vi "Test Save Animated GIF (Memory).vi"(8 "error in (no error)":errorcluster) -> (0 "error out":errorcluster, 3 "Pass?":bool)   [LabVIEW 2020]
uses:
  G-Image/Image IO/Controls/Dither Type.ctl
  G-Image/G-Image.lvlib
  0f1b1910-5d7c-4507-bdef-12e0c9c3451f.vi
  G-Image/Image IO/Polymorphic VIs/Save Animated GIF Image (Memory).vi
  G-Image/Image IO/Polymorphic VIs/Load Animated GIF Image (Memory).vi
panel:
  out "Waveform Chart":cluster{dbl, dbl}(graph)={-0.06975647374412564, 0.4806308479691592}
  out "Array":cluster{string, "new picture":picture}[](array[cluster])
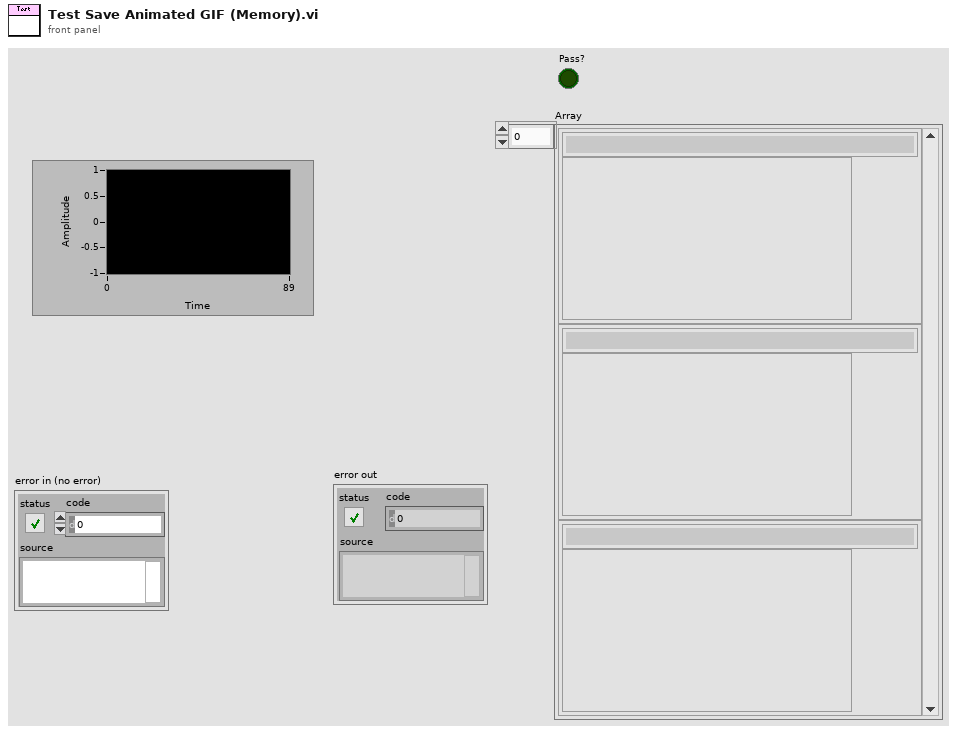
[diagram p1: front panel]
types:
  T1 = typedef "G-Image.lvlib/Dither Type.ctl" = enum32{"None", "Floyd-Steinberg"}
  T2 = typedef "imagedata.ctl" = cluster{"image type":i32, "image depth":i32, "image":u8[], "mask":u8[], "colors":u32[], "Rectangle":cluster{"left":i16, "top":i16, "right":i16, "bottom":i16}}
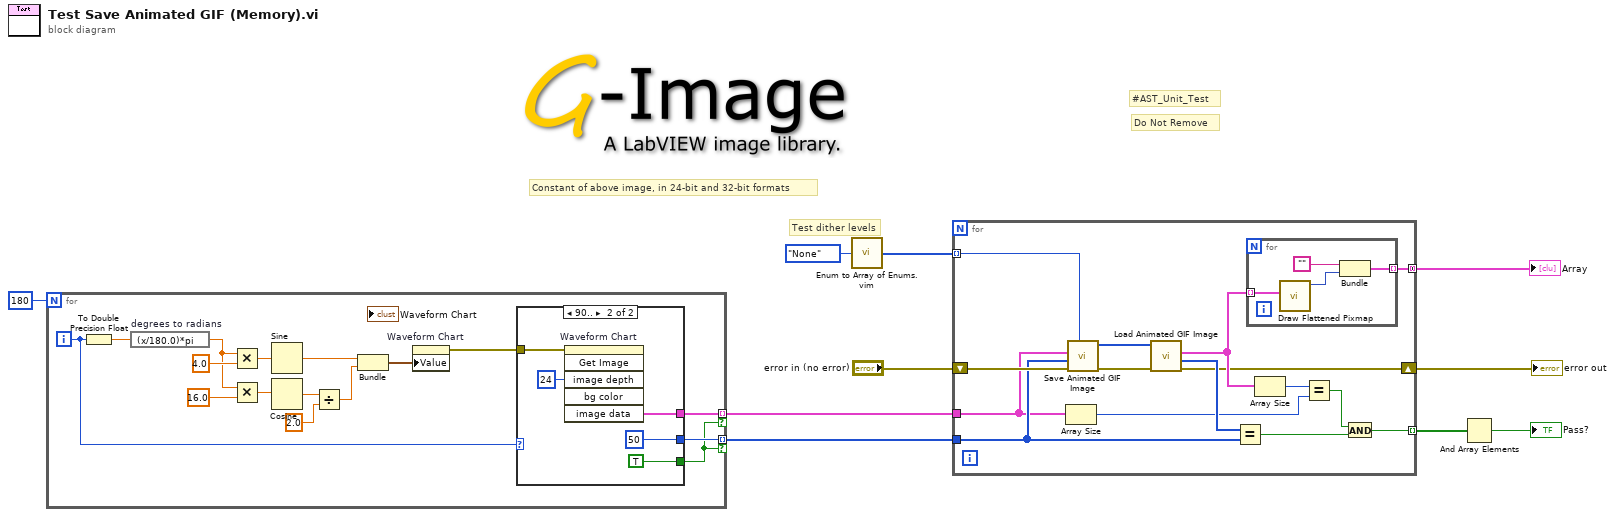
[diagram p0: block diagram]
diagram:
  # "Test dither levels"
  # "Constant of above image, in 24-bit and 32-bit formats"
  # "Do Not Remove"
  # "#AST_Unit_Test"
  n1 = for {
    N: 180 -> [_]
    tunnel: [w26] -> w4 mode=indexing if=w11
    tunnel: [w13] -> w3 mode=indexing if=w11
    i -> [w12]
    n2 = To Double Precision Float(number=w12) -> (double precision float=w23:dbl)
    n3 = expression code="(x/180.0)*pi" "degrees to radians"(w23) -> (w18:dbl)
    n4 = Multiply(x=w18, y=4.0) -> (x*y=w21:dbl)
    n5 = Multiply(x=w18, y=16.0) -> (x*y=w16:dbl)
    n6 = Sine(x=w21) -> (sin(x)=w20:dbl)
    n7 = Cosine(x=w16) -> (cos(x)=w19:dbl)
    n8 = Divide(x=w19, y=2.0) -> (x/y=w15:dbl)
    n9 = Bundle(w20, w15) -> (w22:cluster{dbl, dbl})  [unwired: 1 in]
    n10 = property on="Waveform Chart" class="WFChart (strict)"("Value"=w22) -> (error out=w25:errorcluster)  [unwired: 2 in, 1 out]
    n11 = case shown="90.." w12 {
      tunnel: [_ w30] -> w26
      tunnel: w25 -> [_ w29]
      tunnel: [_ 50] -> w13
      tunnel: [_ TRUE] -> w11
      frame Default {
      }
      frame 90.. {
        n12 = invoke on="Waveform Chart" class="WFChart (strict)" method="Get Image"(error in=w29, "image depth"=24 ("Image Depth")) -> ("image data"=w30:T2)  [unwired: 4 in, 5 out]
      }
    }
  }
  n13 = call "Enum to Array of Enums.vim"("enum"=Dither_Type."None" ("Dither (None)")) -> ("array of enums"=w6:T1[])
  n14 = for {
    shift-right: [w32] -> w8
    shift-left: "error in (no error)" -> [w46]
    tunnel: [w43] -> w9 mode=concatenating
    tunnel: w6 -> [w42] mode=indexing
    tunnel: w4 -> [w39]
    tunnel: w3 -> [w40]
    tunnel: [w33] -> w2 mode=indexing
    n15 = Array Size(array=w39) -> (size(s)=w36:i32)
    n16 = call-poly "Save Animated GIF Image.vi"("Dither (None)"=w42, "error in (no error)"=w46, "Delays"=w40, "Frames"=w39) -> ("error out"=w44:errorcluster, "Encoded Image"=w45:u8[])  [unwired: 6 in]
    n17 = call-poly "Load Animated GIF Image.vi"("error in (no error)"=w44, "Encoded Image"=w45) -> ("error out"=w32:errorcluster, "Delays"=w41:i32[], "Frames"=w38:T2[])  [unwired: 7 in]
    n18 = Equal?(x=w41, y=w40) -> (x = y?=w34:bool)
    n19 = for {
      tunnel: [w49] -> w43 mode=indexing
      tunnel: w38 -> [w48] mode=indexing
      n20 = call <vilib>:"Draw Flattened Pixmap.vi"("image data"=w48) -> ("new picture"=w50:picture)  [unwired: 8 in]
      n21 = Bundle("", "new picture"=w50) -> (w49:cluster{string, "new picture":picture})  [unwired: 1 in]
    }
    n22 = Array Size(array=w38) -> (size(s)=w37:i32)
    n23 = Equal?(x=w37, y=w36) -> (x = y?=w35:bool)
    n24 = And(x=w35, y=w34) -> (x .and. y?=w33:bool)
  }
  "error out" <- w8
  "Array" <- w9
  n25 = And Array Elements(Boolean array=w2) -> (logical AND=→"Pass?":bool)
